vi "FreeUnpackedFields.vi"(8 "error in (no error)":errorcluster, 11 "Unpacked Fields ID":T1) -> (0 "error out":errorcluster)   [LabVIEW 2019, in "Template Server.lvlib" / "gprc-lvsupport.lvlib"]
uses:
  gprc-lvsupport.lvlib
  typeDefs/grpcId.ctl
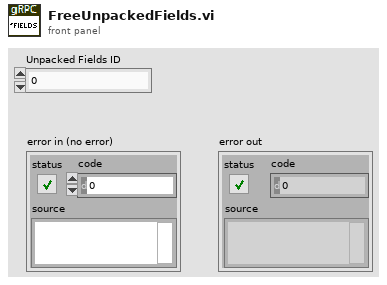
[diagram p1: front panel]
types:
  T1 = typedef "Template Server.lvlib/gprc-lvsupport.lvlib/grpcId.ctl" = u64
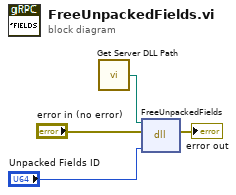
[diagram p0: block diagram]
diagram:
  n1 = call "Get Server DLL Path.vi"() -> ("Server dll path"=w3:path)
  n2 = dll-call lib="?" fn="FreeUnpackedFields"(path in=w3, error in="error in (no error)", "serializationId"="Unpacked Fields ID") -> (error out=→"error out":errorcluster)  [unwired: 3 in, 1 out]
